vi "sub_solve.vi"(10 "solver (in)":cluster{"solved":bool, "values":string[]}[][](array[cluster])=[[{"solved"=TRUE, "values"=["7"]}, {"solved"=TRUE, "values"=["5"]}, {"solved"=FALSE, "values"=["2", "5", "8"]}, {"solved"=FALSE, "values"=["8", "9"]}, {"solved"=FALSE, "values"=["1", "5", "8", "9"]}, {"solved"=TRUE, "values"=["3"]}, {"solved"=TRUE, "values"=["6"]}, {"solved"=TRUE, "values"=["4"]}, {"solved"=FALSE, "values"=["1", "2", "9"]}], [{"solved"=TRUE, "values"=["6"]}, {"solved"=TRUE, "values"=["9"]}, {"solved"=TRUE, "values"=["4"]}, {"solved"=TRUE, "values"=["2"]}, {"solved"=FALSE, "values"=["1", "8"]}, {"solved"=TRUE, "values"=["7"]}, {"solved"=FALSE, "values"=["1", "8"]}, {"solved"=TRUE, "values"=["5"]}, {"solved"=TRUE, "values"=["3"]}], [{"solved"=TRUE, "values"=["3"]}, {"solved"=FALSE, "values"=["2", "5"]}, {"solved"=TRUE, "values"=["1"]}, {"solved"=FALSE, "values"=["4", "8", "9"]}, {"solved"=FALSE, "values"=["5", "6", "8", "9"]}, {"solved"=FALSE, "values"=["5", "6"]}, {"solved"=FALSE, "values"=["8", "9"]}, {"solved"=TRUE, "values"=["7"]}, {"solved"=FALSE, "values"=["2", "9"]}], [{"solved"=TRUE, "values"=["5"]}, {"solved"=TRUE, "values"=["1"]}, {"solved"=TRUE, "values"=["7"]}, {"solved"=TRUE, "values"=["6"]}, {"solved"=TRUE, "values"=["2"]}, {"solved"=TRUE, "values"=["8"]}, {"solved"=TRUE, "values"=["3"]}, {"solved"=TRUE, "values"=["9"]}, {"solved"=TRUE, "values"=["4"]}], [{"solved"=TRUE, "values"=["2"]}, {"solved"=TRUE, "values"=["3"]}, {"solved"=TRUE, "values"=["9"]}, {"solved"=TRUE, "values"=["7"]}, {"solved"=TRUE, "values"=["4"]}, {"solved"=TRUE, "values"=["1"]}, {"solved"=TRUE, "values"=["5"]}, {"solved"=TRUE, "values"=["6"]}, {"solved"=TRUE, "values"=["8"]}], [{"solved"=TRUE, "values"=["4"]}, {"solved"=TRUE, "values"=["8"]}, {"solved"=TRUE, "values"=["6"]}, {"solved"=TRUE, "values"=["5"]}, {"solved"=TRUE, "values"=["3"]}, {"solved"=TRUE, "values"=["9"]}, {"solved"=TRUE, "values"=["2"]}, {"solved"=TRUE, "values"=["1"]}, {"solved"=TRUE, "values"=["7"]}], [{"solved"=TRUE, "values"=["1"]}, {"solved"=FALSE, "values"=["2", "4", "5"]}, {"solved"=FALSE, "values"=["2", "3", "5"]}, {"solved"=FALSE, "values"=["3", "9"]}, {"solved"=TRUE, "values"=["7"]}, {"solved"=FALSE, "values"=["2", "5", "6"]}, {"solved"=FALSE, "values"=["4", "9"]}, {"solved"=TRUE, "values"=["8"]}, {"solved"=FALSE, "values"=["5", "9"]}], [{"solved"=TRUE, "values"=["9"]}, {"solved"=TRUE, "values"=["6"]}, {"solved"=FALSE, "values"=["3", "5"]}, {"solved"=FALSE, "values"=["3", "8"]}, {"solved"=FALSE, "values"=["5", "8"]}, {"solved"=TRUE, "values"=["4"]}, {"solved"=FALSE, "values"=["1", "7"]}, {"solved"=TRUE, "values"=["2"]}, {"solved"=FALSE, "values"=["1", "5"]}], [{"solved"=TRUE, "values"=["8"]}, {"solved"=TRUE, "values"=["7"]}, {"solved"=FALSE, "values"=["2", "5"]}, {"solved"=TRUE, "values"=["1"]}, {"solved"=FALSE, "values"=["5", "9"]}, {"solved"=FALSE, "values"=["2", "5"]}, {"solved"=FALSE, "values"=["4", "9"]}, {"solved"=TRUE, "values"=["3"]}, {"solved"=TRUE, "values"=["6"]}]] caption="solver array", 11 "puzzle (in)":string[][](array[string])=[["", "1", "", "", "", "", "", ""], ["", "", "6", "", "", "", "6", ""], ["", "", "", "", "6", "", "", ""], ["", "", "", "", "", "", "", ""], ["2", "", "", "6", "7", "", "", "9"], ["", "6", "", "", "", "", "", ""], ["", "6", "", "", "4", "", "", ""], ["", "", "", "", "", "", "", ""], ["", "3", "", "", "2", "", "", "3"]]) -> (2 "solver (out)":cluster{"solved":bool, "values":string[]}[][](array[cluster]))   [LabVIEW 2018]
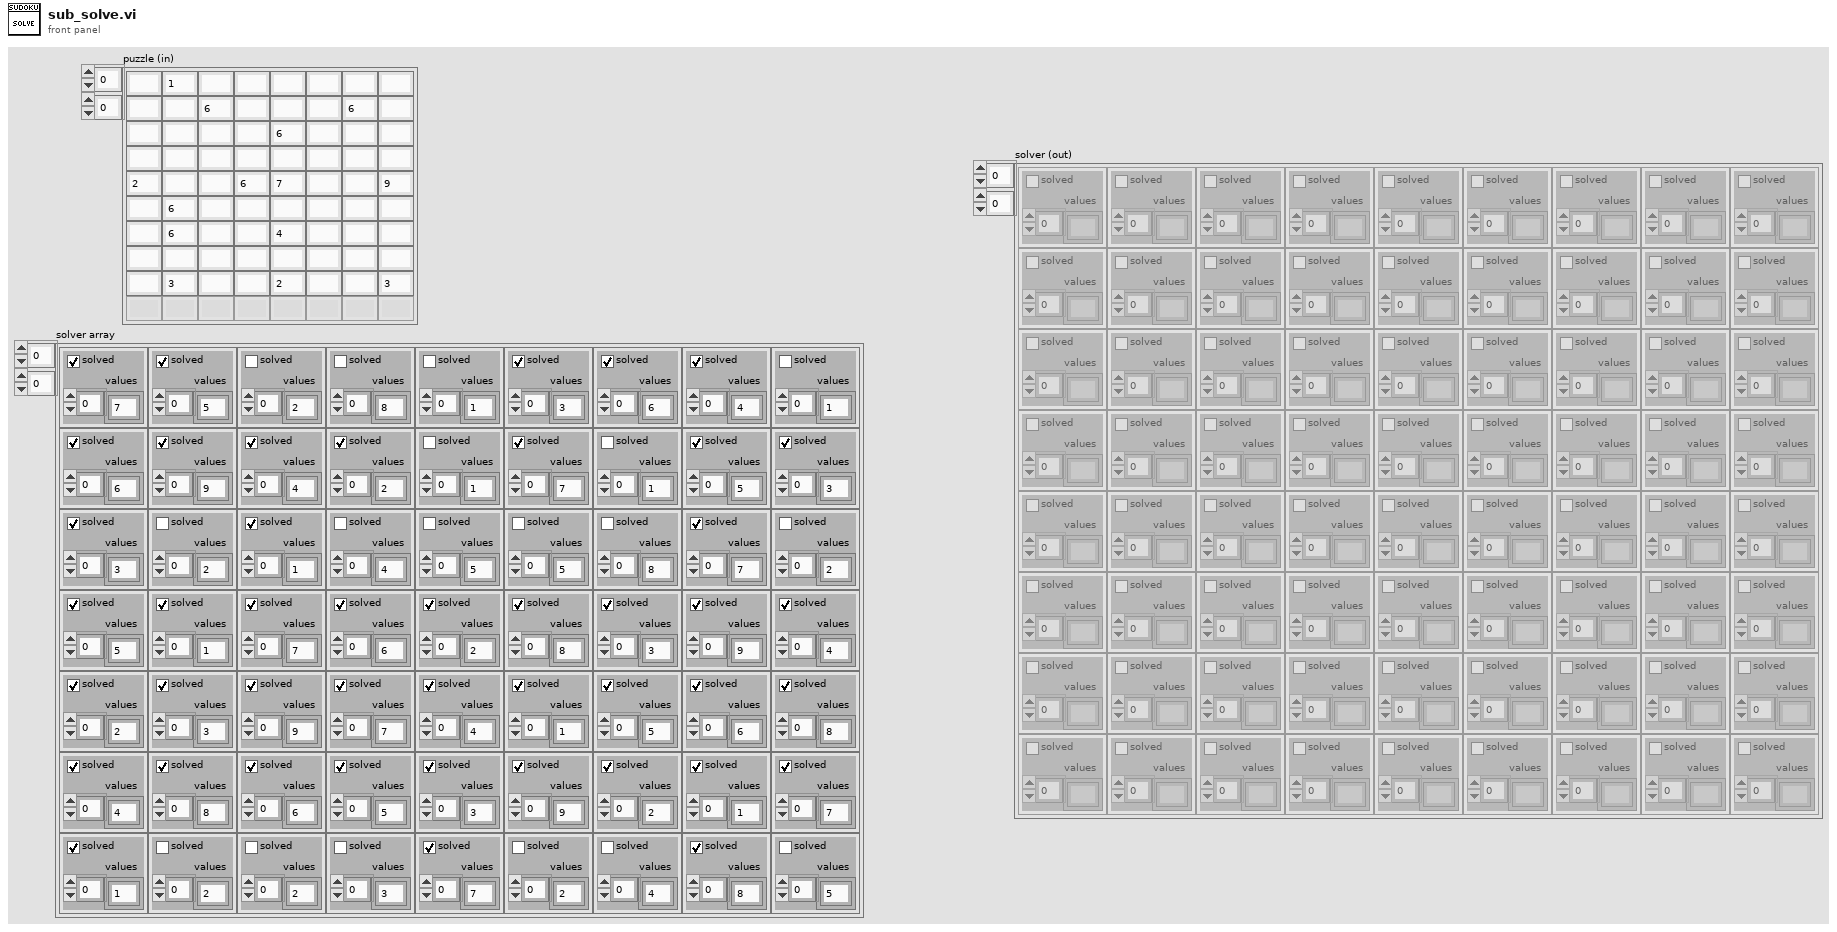
[diagram p1: front panel]
types:
  T1 = typedef "cell.ctl" = cluster{"solved":bool, "values":string[]}
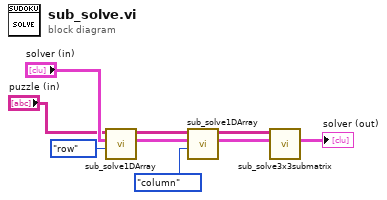
[diagram p0: block diagram]
diagram:
  n1 = call "sub_solve1DArray.vi"("type"=enum16{"row", "column"}."row", "solver (in)"="solver (in)", "puzzle"="puzzle (in)") -> ("solver (out)"=w7:T1[][], "puzzle (out)"=w2:string[][])  [unwired: 7 in]
  n2 = call "sub_solve1DArray.vi"("type"=enum16{"row", "column"}."column", "solver (in)"=w7, "puzzle"=w2) -> ("solver (out)"=w5:T1[][], "puzzle (out)"=w1:string[][])  [unwired: 7 in]
  n3 = call "sub_solve3x3submatrix.vi"("solver (in)"=w5, "puzzle (in)"=w1) -> ("solver (out)"=→"solver (out)":cluster{"solved":bool, "values":string[]}[][])  [unwired: 9 in]
